vi "Helmholtzresonansformel.vi"() -> ()   [LabVIEW 2014]
panel:
  out "output variable":dbl
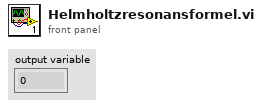
[diagram p1: front panel]
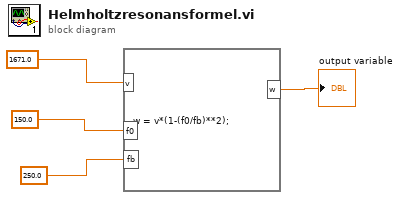
[diagram p0: block diagram]
diagram:
  n1 = formula code="w = v*(1-(f0/fb)**2);"("v"=1671.0 ("input variable"), "f0"=150.0 ("input variable"), "fb"=250.0 ("input variable")) -> ("w"=→"output variable":dbl)
